vi "Data Types.vi"(8 "error in (no error)":errorcluster, 9 "Operation":enum16{"Get", "Set"}(ring), 11 "Data Types":string[](array[string])) -> (0 "error out":errorcluster, 3 "Data Types (out)":string[](array[string]))   [LabVIEW 2017, in "WebServiceImporter.lvlib" / "ProxyDll Generator.lvlib"]
uses:
  <vilib>/Platform/WebService/ProxyDll Generator/ProxyDll Generator.lvlib
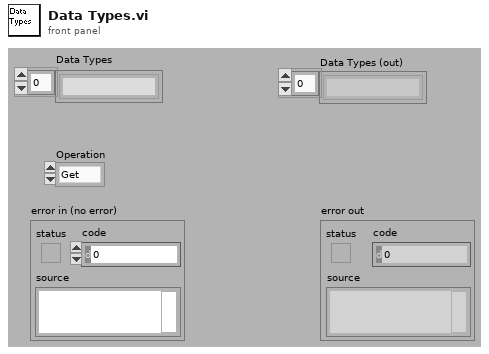
[diagram p1: front panel]
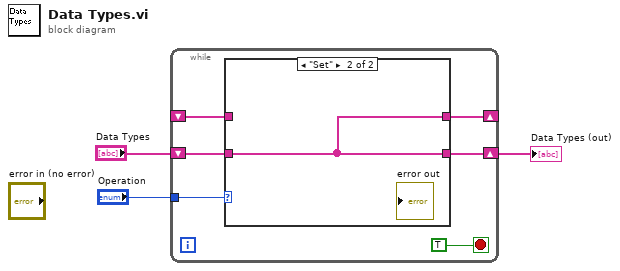
[diagram p0: block diagram]
diagram:
  n1 = while {
    tunnel: "Operation" -> [w8]
    shift-right: [w6] -> w1
    shift-left: "Data Types" -> [w7]
    shift-right: [w5] -> _
    shift-left: _ -> [w4]
    stop <- TRUE stop-if-true
    n2 = case shown="\"Set\"" w8 {
      tunnel: w7 -> [_ w11]
      tunnel: [w10 w11] -> w6
      tunnel: [w10 w11] -> w5
      tunnel: w4 -> [w10 _]
      frame "Get", Default {
      }
      frame "Set" {
      }
    }
  }
  "Data Types (out)" <- w1
